vi "VG_VCellMax30_P.vi"() -> ()   [LabVIEW 2020]
panel:
  out "VCellMax30":dbl
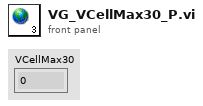
[diagram p1: front panel]
diagram:
